vi "ProdaNG.File.ExportToFile.vi"(8 "error in (no error)":errorcluster) -> (0 "error out":errorcluster, 2 "FileContent":T1)   [LabVIEW 2016]
uses:
  ProdaNG.File.Sequence.ctl
  ProdaNG.Tree.Fglb.Value.ctl
  ProdaNG.File.Step.ctl
  ProdaNG.Configurator.Glb.vi
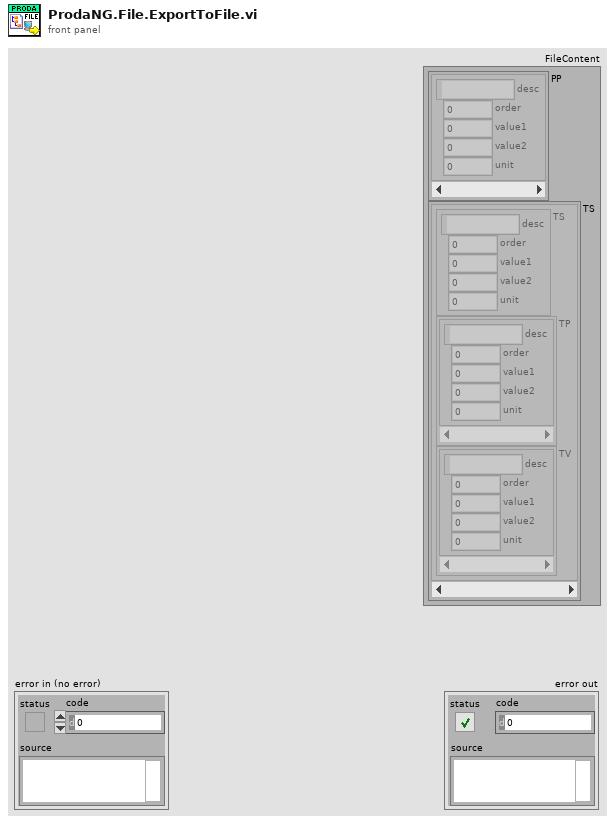
[diagram p1: front panel]
types:
  T1 = typedef "ProdaNG.File.Sequence.ctl" = cluster{"PP":T2[], "TS":T3[]}
  T2 = typedef "ProdaNG.Tree.Fglb.Value.ctl" = cluster{"desc":string, "order":i32, "value1":dbl, "value2":dbl, "unit":i32}
  T3 = typedef "ProdaNG.File.Step.ctl" = cluster{"TS":T2, "TP":T2[], "TV":T2[]}
  T4 = typedef "ProdaNG.ProcessStepParam.ctl" = cluster{"i_id":i32, "processStepId":i32, "unitId":i32, "contentId":string, "previewId":string, "value":dbl, "valueText":string, "paramSequence":i32, "history":i32, "mdReason":string, "mdUser":string, "mdTime":string, "description":string}
  T5 = typedef "ProdaNG.TestStep.ctl" = cluster{"i_id":i32, "processStepId":i32, "testSequence":i32, "testOrder":i32, "mdReason":string, "mdUser":string, "mdTime":string, "description":string}
  T6 = typedef "ProdaNG.TestStepParam.ctl" = cluster{"i_id":i32, "testStepId":i32, "unitId":i32, "contentId":string, "previewId":string, "value":dbl, "valueText":string, "paramSequence":i32, "history":i32, "mdReason":string, "mdUser":string, "mdTime":string, "description":string}
  T7 = typedef "ProdaNG.TestValue.ctl" = cluster{"i_id":i32, "testStepId":i32, "releaseId":i32, "unitId":i32, "contentId":string, "previewId":string, "maximum":dbl, "minimum":dbl, "valueText":string, "testValueSequence":i32, "history":i32, "mdReason":string, "mdUser":string, "mdTime":string, "description":string}
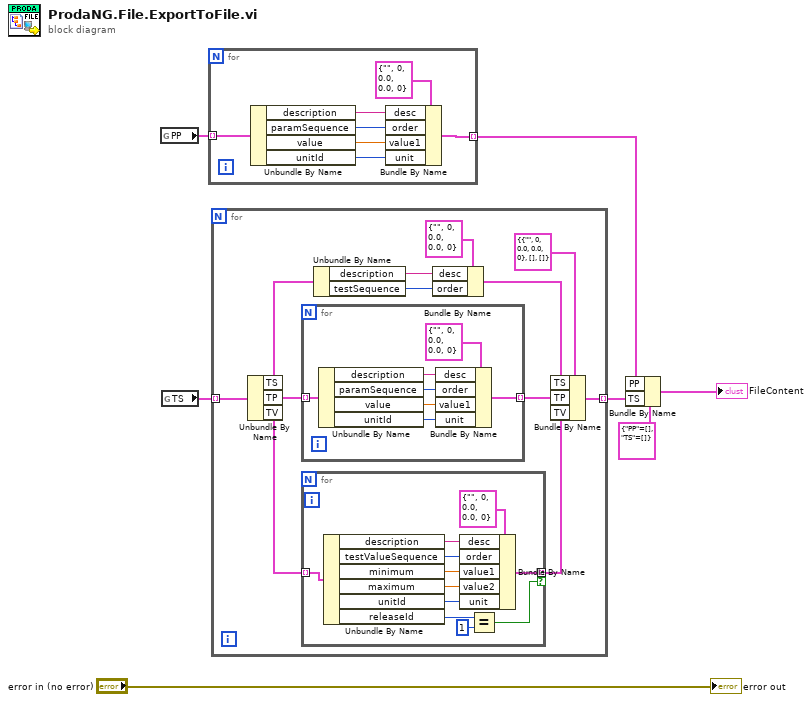
[diagram p0: block diagram]
diagram:
  n1 = global read "ProdaNG.Configurator.Glb.vi" "PP"() -> (w5:T4[])
  n2 = global read "ProdaNG.Configurator.Glb.vi" "TS"() -> (w4:cluster{"TS":T5, "TP":T6[], "TV":T7[]}[])
  n3 = for {
    tunnel: w5 -> [w13] mode=indexing
    tunnel: [w11] -> w1 mode=indexing
    n4 = Unbundle By Name(w13) -> ("description"=w12:string, "paramSequence"=w10:i32, "value"=w8:dbl, "unitId"=w9:i32)
    n5 = Bundle By Name(cluster=T2 {"desc"="", "order"=0, "value1"=0.0, "value2"=0.0, "unit"=0} ("Element values"), "desc"=w12, "order"=w10, "value1"=w8, "unit"=w9) -> (w11:T2)
  }
  n6 = for {
    tunnel: w4 -> [w26] mode=indexing
    tunnel: [w15] -> w3 mode=indexing
    n7 = Unbundle By Name(w26) -> ("TS"=w20:T5, "TP"=w25:T6[], "TV"=w22:T7[])
    n8 = for {
      tunnel: w25 -> [w39] mode=indexing
      tunnel: [w38] -> w23 mode=indexing
      n9 = Unbundle By Name(w39) -> ("description"=w41:string, "paramSequence"=w42:i32, "value"=w44:dbl, "unitId"=w43:i32)
      n10 = Bundle By Name(cluster=T2 {"desc"="", "order"=0, "value1"=0.0, "value2"=0.0, "unit"=0} ("Element values"), "desc"=w41, "order"=w42, "value1"=w44, "unit"=w43) -> (w38:T2)
    }
    n11 = for {
      tunnel: w22 -> [w32] mode=indexing
      tunnel: [w31] -> w21 mode=indexing if=w27
      n12 = Unbundle By Name(w32) -> ("description"=w34:string, "testValueSequence"=w35:i32, "minimum"=w37:dbl, "maximum"=w30:dbl, "unitId"=w36:i32, "releaseId"=w29:i32)
      n13 = Bundle By Name(cluster=T2 {"desc"="", "order"=0, "value1"=0.0, "value2"=0.0, "unit"=0} ("Element values"), "desc"=w34, "order"=w35, "value1"=w37, "value2"=w30, "unit"=w36) -> (w31:T2)
      n14 = Equal?(x=w29, y=1) -> (x = y?=w27:bool)
    }
    n15 = Unbundle By Name(w20) -> ("description"=w18:string, "testSequence"=w17:i32)
    n16 = Bundle By Name(cluster=T2 {"desc"="", "order"=0, "value1"=0.0, "value2"=0.0, "unit"=0} ("TS"), "desc"=w18, "order"=w17) -> (w16:T2)
    n17 = Bundle By Name(cluster=T3 {"TS"={"desc"="", "order"=0, "value1"=0.0, "value2"=0.0, "unit"=0}, "TP"=[], "TV"=[]} ("Step"), "TS"=w16, "TP"=w23, "TV"=w21) -> (w15:T3)
  }
  n18 = Bundle By Name(cluster=T1 {"PP"=[], "TS"=[]} ("FileContent"), "PP"=w1, "TS"=w3) -> (→"FileContent":T1)
  "error out" <- "error in (no error)"
